vi "Cleanup Host Stream.vi"(8 "error in (no error)":errorcluster, 11 "Refs":T1) -> (0 "error out":errorcluster)   [LabVIEW 2019, in "CAN Streaming Support Workspace Shared.lvlib"]
uses:
  CAN Streaming Support Workspace Shared.lvlib
  Types/Host Stream API Refs.ctl
  <vilib>/xnet/xnet.llb/XNET CAN Comm.ctl
  <vilib>/xnet/xnet.llb/XNET CAN Comm State.ctl
  <vilib>/xnet/xnet.llb/XNET CAN Last Err.ctl
  <vilib>/xnet/xnet.llb/XNET Frame CAN.ctl
  <vilib>/xnet/xnet.llb/XNET Frame Type CAN.ctl
  <vilib>/ErrorRing/Error Ring.xnode
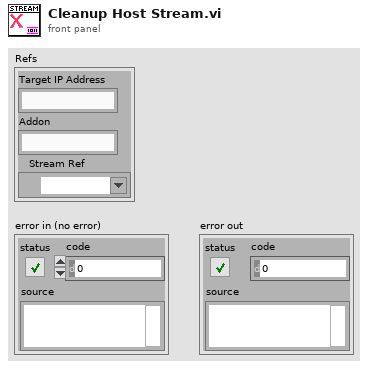
[diagram p1: front panel]
types:
  T1 = typedef "CAN Streaming Support Workspace Shared.lvlib/Host Stream API Refs.ctl" = cluster{"Target IP Address":string, "Addon":string, "Stream Ref":refnum<k21>}
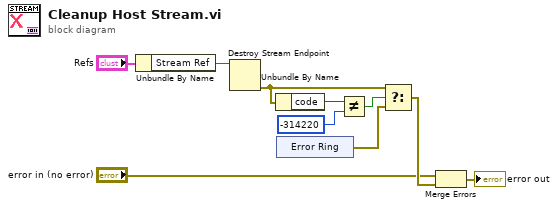
[diagram p0: block diagram]
diagram:
  n1 = Unbundle By Name("Refs") -> ("Stream Ref"=w10:refnum<k21>)
  n2 = Destroy Stream Endpoint(11:w10) -> (0:w8:errorcluster)  [unwired: 1 in]
  n3 = Unbundle By Name(w8) -> ("code"=w5:i32)
  n4 = xnode "Error Ring"() -> ("error out"=w9:errorcluster)
  n5 = Not Equal?(x=w5, y=-314220) -> (x != y?=w7:bool)
  n6 = Select(t=w8, s=w7, f=w9) -> (s? t:f=w3:errorcluster)
  n7 = Merge Errors("error in (no error)", w3) -> (→"error out":errorcluster)
